vi "Try Match Response.vi"(8 "error in":errorcluster, 10 "ICAN CC Frame":refnum<class "ICAN CC Frame.lvclass">, 11 "Segmented Upload Transfer":refnum<class "Segmented Upload Transfer.lvclass">) -> (0 "error out":errorcluster, 2 "Match":bool, 3 "SDO Transfer":refnum<class "SDO Transfer.lvclass">)   [LabVIEW 2020, in "CANopen.lvlib" / "SDO Manager.lvlib" / "Segmented Upload Transfer.lvclass"]
uses:
  Segmented Upload Transfer.lvclass
  SDO Transfer/SDO Transfer.lvclass
  HAL/Source/Interfaces/ICAN CC Frame/ICAN CC Frame.lvclass
  Segmented Upload Transfer.lvclass/Segmented Upload Transfer.ctl
  D:/git/CANopen-LabVIEW/source/SDO/SDO Manager/SDO Transfer/SDO Transfer.lvclass
  D:/git/CANopen-LabVIEW/source/SDO/SDO Manager/Segmented Upload Transfer/Segmented Upload Transfer.lvclass
  CANopen Message/CANopen Message.lvclass
  SDO Transfer/SDO abort code.ctl
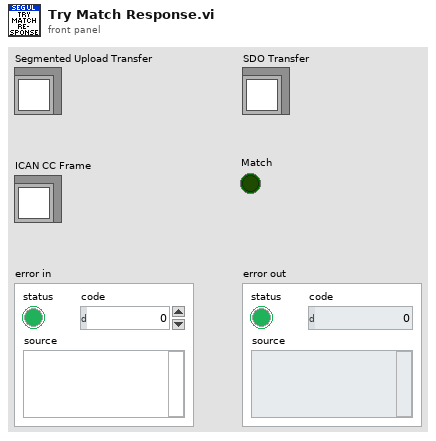
[diagram p1: front panel]
types:
  T1 = typedef "CANopen.lvlib/SDO Manager.lvlib/SDO Transfer.lvclass/SDO abort code.ctl" = u32
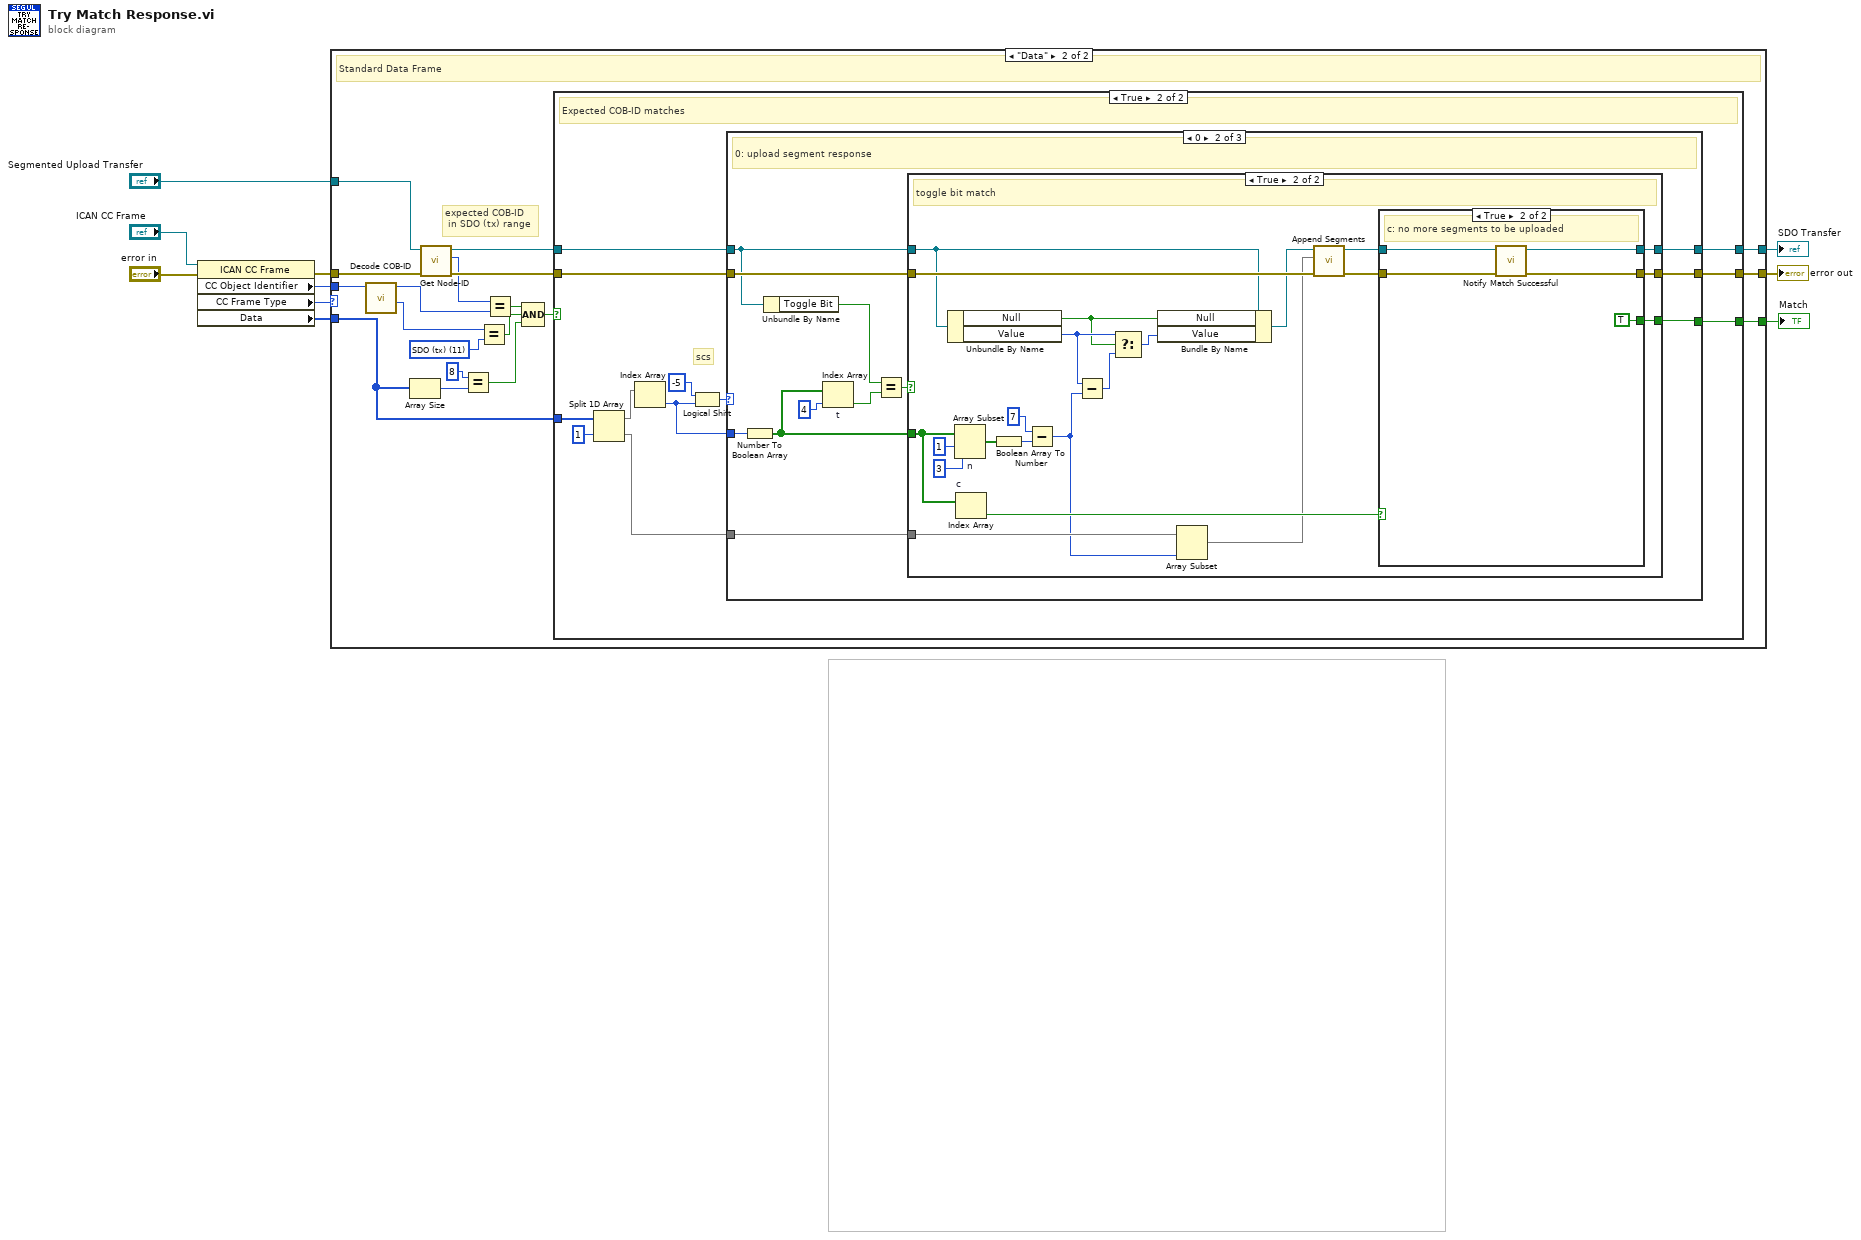
[diagram p0: block diagram]
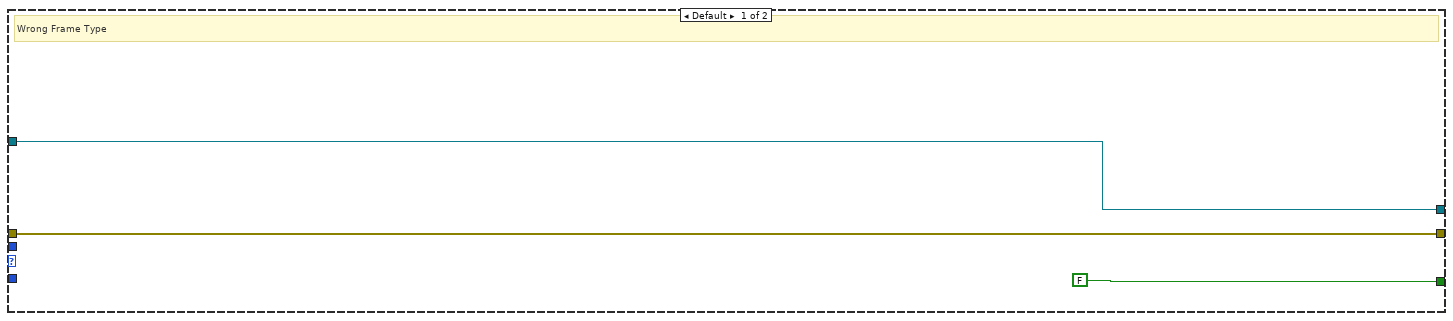
[diagram p2: hidden frame]
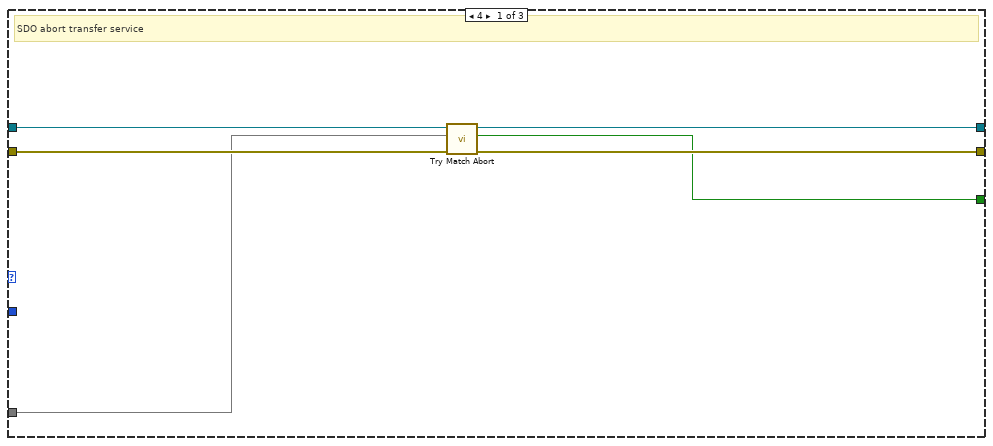
[diagram p4: hidden frame]
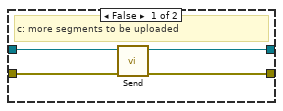
[diagram p6: hidden frame]
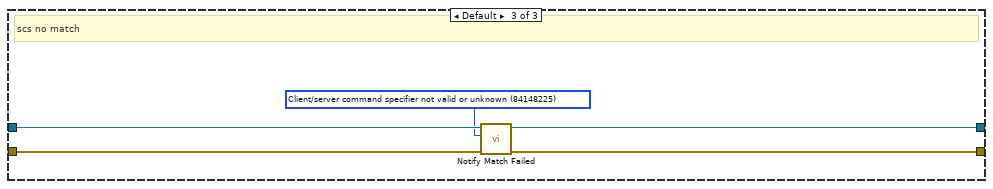
[diagram p7: hidden frame]
diagram:
  n1 = property class="ICAN CC Frame"(reference="ICAN CC Frame", error in="error in") -> (error out=w8:errorcluster, "CC Object Identifier"=w3:u32, "CC Frame Type"=w1:enum8{"Data", "Remote", "Error", "Overload"}, "Data"=w2:u8[])  [unwired: 1 out]
  n2 = case shown="\"Data\"" w1 {
    tunnel: w8 -> [w12 w32]
    tunnel: "Segmented Upload Transfer" -> [w11 w31]
    tunnel: [w11 w28] -> w6
    tunnel: [w12 w27] -> w5
    tunnel: [FALSE w26] -> w4
    tunnel: w3 -> [_ w25]
    tunnel: w2 -> [_ w14]
    frame Default {
      # "Wrong Frame Type"
    }
    frame "Data" {
      w22 = u8 11 items=["NMT"=0, "EMCY/SYNC"=1, "TIME"=2, "PDO1 (tx)"=3, "PDO1 (rx)"=4, "PDO2 (tx)"=5, "PDO2 (rx)"=6, "PDO3 (tx)"=7, "PDO3 (rx)"=8, "PDO4 (tx)"=9, "PDO4 (rx)"=10, "SDO (tx)"=11, "SDO (rx)"=12, "NMT error control"=14] ("Function Code")
      # "expected COB-ID\n in SDO (tx) range"
      # "Standard Data Frame"
      n3 = call "Decode COB-ID.vi"("COD-ID"=w25) -> ("Function Code"=w21:u8, "Node-ID"=w24:u8)  [unwired: 9 in]
      n4 = Array Size(array=w14) -> (size(s)=w20:i32)
      n5 = call "Get Node-ID.vi"("error in"=w32, "SDO Transfer in"=w31) -> ("error out"=w29:errorcluster, "Node-ID"=w23:u8, "SDO Transfer out"=w30:refnum<class "Segmented Upload Transfer.lvclass">)  [unwired: 7 in]
      n6 = Equal?(x=8, y=w20) -> (x = y?=w15:bool)
      n7 = Equal?(x=w21, y=w22) -> (x = y?=w16:bool)
      n8 = Equal?(x=w23, y=w24) -> (x = y?=w17:bool)
      n9 = Compound Arithmetic op=AND(w17, w16, w15) -> (w18:bool)
      n10 = case shown="True" w18 {
        tunnel: w30 -> [w34 w45]
        tunnel: w29 -> [w33 w44]
        tunnel: [w34 w41] -> w28
        tunnel: [w33 w42] -> w27
        tunnel: w14 -> [_ w39]
        tunnel: [_ w40] -> w26
        frame False {
        }
        frame True {
          # "scs"
          # "Expected COB-ID matches"
          n11 = Split 1D Array(array=w39, index=1) -> (first subarray=w37:u8[], second subarray=w35:u8[])
          n12 = Index Array(array=w37) -> (element=w36:u8)  [unwired: 1 in]
          n13 = Logical Shift(y=i16 -5, x=w36) -> (x << y=w43:u8)
          n14 = case shown="0" w43 {
            tunnel: w45 -> [w51 w60 w100]
            tunnel: w44 -> [w52 w64 w102]
            tunnel: [w50 w62 w99] -> w41
            tunnel: [w49 w63 w101] -> w42
            tunnel: [w48 w61 _] -> w40
            tunnel: w35 -> [w47 w54 _]
            tunnel: w36 -> [_ w53 _]
            frame 4 {
              # "SDO abort transfer service"
              n15 = call "Try Match Abort.vi"("error in"=w52, "Data"=w47, "SDO Transfer in"=w51) -> ("error out"=w49:errorcluster, "Success"=w48:bool, "SDO Transfer out"=w50:refnum<class "Segmented Upload Transfer.lvclass">)  [unwired: 6 in]
            }
            frame 0 {
              # "0: upload segment response"
              n16 = Number To Boolean Array(number=w53) -> (Boolean array=w55:bool[])
              n17 = Unbundle By Name(w60) -> ("Toggle Bit"=w59:bool)
              n18 = Index Array "t"(array=w55, index=4 ("t")) -> (element=w56:bool)
              n19 = Equal?(x=w59, y=w56) -> (x = y?=w58:bool)
              n20 = case shown="True" w58 {
                tunnel: w64 -> [w65 w88]
                tunnel: [w65 w87] -> w63
                tunnel: [w66 w86] -> w62
                tunnel: [_ w85] -> w61
                tunnel: w54 -> [_ w84]
                tunnel: w60 -> [w66 w83]
                tunnel: w55 -> [_ w73]
                frame False {
                  # "#todo: sdo abort on toggle bit mismatch or just do nothing?"
                  # "toggle bit mismatch"
                }
                frame True {
                  # "toggle bit match"
                  n21 = Unbundle By Name(w83) -> ("Null"=w79:bool, "Value"=w82:u32)
                  n22 = Array Subset "n"(array=w73, index=1 ("n"), length=3) -> (w77:bool[])
                  n23 = Index Array "c"(array=w73) -> (element=w78:bool)  [unwired: 1 in]
                  n24 = Boolean Array To Number(Boolean array=w77) -> (number=w74:u32)
                  n25 = Subtract(x=u32 7, y=w74) -> (x-y=w67:u32)
                  n26 = Subtract(x=w82, y=w67) -> (x-y=w81:u32)
                  n27 = Select(t=w82, s=w79, f=w81) -> (s? t:f=w80:u32)
                  n28 = Bundle By Name(cluster=w83, "Null"=w79, "Value"=w80) -> (w70:refnum<class "Segmented Upload Transfer.lvclass">)
                  n29 = Array Subset(array=w84, length=w67) -> (w68:u8[])  [unwired: 1 in]
                  n30 = call "Append Segments.vi"("error in"=w88, "Segments"=w68, "Segmented Upload Transfer in"=w70) -> ("error out"=w71:errorcluster, "Segmented Upload Transfer out"=w69:refnum<class "Segmented Upload Transfer.lvclass">)  [unwired: 7 in]
                  n31 = case shown="True" w78 {
                    tunnel: w71 -> [w91 w96]
                    tunnel: [w90 w95] -> w87
                    tunnel: [w92 w93] -> w86
                    tunnel: [_ TRUE] -> w85
                    tunnel: w69 -> [w89 w94]
                    frame False {
                      # "c: more segments to be uploaded"
                      n32 = call-dynamic "Send.vi"("error in"=w91, "Segmented Upload Transfer"=w89) -> ("error out"=w90:errorcluster, "Segmented Upload Transfer"=w92:refnum<class "Segmented Upload Transfer.lvclass">)  [unwired: 8 in]
                    }
                    frame True {
                      # "c: no more segments to be uploaded"
                      n33 = call "Notify Match Successful.vi"("error in"=w96, "SDO Transfer in"=w94) -> ("error out"=w95:errorcluster, "SDO Transfer out"=w93:refnum<class "Segmented Upload Transfer.lvclass">)  [unwired: 8 in]
                    }
                  }
                }
              }
            }
            frame Default {
              w98 = T1 84148225 items=["Toggle bit not allowed"=84082688, "SDO protocol timed out"=84148224, "Client/server command specifier not valid or unknown"=84148225, "Invalid block size (block mode only)"=84148226, "Invalid sequence number (block mode only)"=84148227, "CRC error (block mode only)"=84148228, "Out of memory"=84148229, "Attempt to read a write only object"=100728833, "Attempt to write a read only object"=100728834, "Object does not exist in the object dictionary"=100794368, "Object cannot be mapped to the PDO"=100925505, "The number and length of the objects to be mapped would exceed PDO length"=100925506, "General parameter incompatibility reason"=100925507, "General internal incompatibility in the device"=100925511, "Access failed due to an hardware error"=101056512, "Data type does not match, length of service parameter does not match"=101122064, "Data type does not match, length of service parameter too high"=101122066, "Data type does not match, length of service parameter too low"=101122067, "Sub-index does not exist"=101253137, "Invalid value for parameter (download only)"=101253168, "Value of parameter written too high (download only)"=101253169, "Value of parameter written too low (download only)"=101253170, "Maximum value is less than minimum value"=101253174, "Resource not available: SDO connection"=101318691, "General error"=134217728, "Data cannot be transferred or stored to the application"=134217760, "Data cannot be transferred or stored to the application because of local control"=134217761, "Data cannot be transferred or stored to the application because of the present device stable"=134217762, "Object dictionary dynamic generation fails or no object dictionary is present (e.g. object dictionary is generated from file and generation fails because of an file error)"=134217763, "No data available"=134217764] ("SDO abort code")
              # "scs no match"
              n34 = call "Notify Match Failed.vi"("error in"=w102, "SDO abort code"=w98, "SDO Transfer in"=w100) -> ("error out"=w101:errorcluster, "SDO Transfer out"=w99:refnum<class "Segmented Upload Transfer.lvclass">)  [unwired: 7 in]
            }
          }
        }
      }
    }
  }
  "SDO Transfer" <- w6
  "error out" <- w5
  "Match" <- w4
